vi "3-1 random controllo se compreso STOP.vi"(1 "control":bool, 2 "low limit":dbl(knob) scale=0.0..10.0 scale format="%.1f", 3 "hight limit":dbl(knob) scale=0.0..10.0 scale format="%.1f", 4 "stop":bool) -> (0 "data out":dbl(knob) scale=0.0..11.0 scale format="%.1f")   [LabVIEW 2012]
doc: "© Copyright M. Ferrari 1999"
panel:
  out "data in":dbl format="%.2f"
  # "Se control = ON, bisogna verificare che il valore sia compreso nei limiti\n                     trasferendo il valore di ingresso diviso per il range ( hight limit-low limit)\n                     in uscita; se il valore  \"data in\"  non rientra nei limiti, oppure \nse control = OFF, non viene effettuato nessun controllo e il valore di ingresso passa direttamente in uscita"
  # "Completare il VI facendo in modo che venga eseguito ciclicamente ogni 2 sec. e che \nl' esecuzione venga terminata nel caso in cui il dato in ingresso (data in) sia il doppio\ndi hight limit, oppure nel caso in cui venga premuto un apposito pulsante \"STOP\" (che \nandrˆ inserito nel pannello di controllo). Inoltre il dato di ingresso ( indicato con data in) \ndovrˆ essere generato automaticamente e risultare un valore casuale compreso fra 1 e 11"
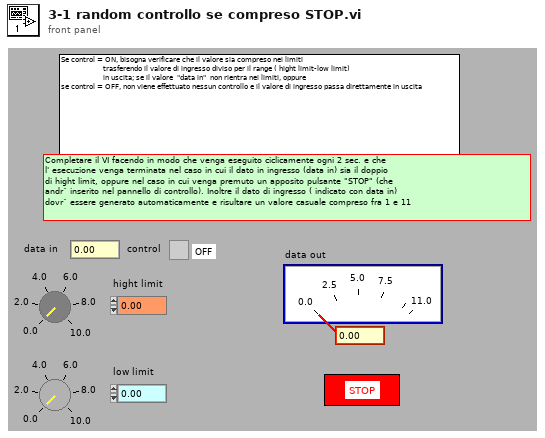
[diagram p1: front panel]
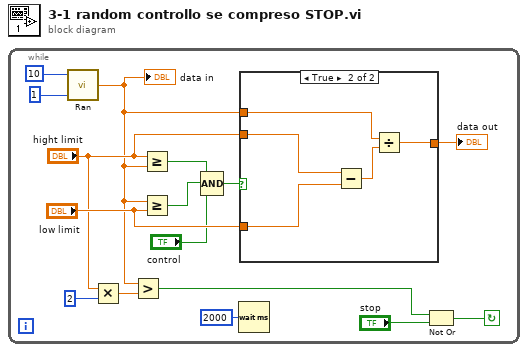
[diagram p0: block diagram]
diagram:
  n1 = while {
    stop <- w2 continue-if-true
    n2 = call "Ran.vi"("offset"=1, "mul fatt"=10) -> ("out num"=w5:dbl)  [unwired: 3 in]
    "data in" <- w5
    n3 = Multiply(x="hight limit", y=2) -> (x*y=w6:dbl)
    n4 = Greater?(x=w5, y=w6) -> (0:w4:bool)
    n5 = Greater Or Equal?(x="hight limit", y=w5) -> (x >= y?=w12:bool)
    n6 = Greater Or Equal?(x=w5, y="low limit") -> (x >= y?=w13:bool)
    n7 = Compound Arithmetic op=AND(w12, w13, "control") -> (w15:bool)
    n8 = Wait (ms)(milliseconds to wait=u32 2000) -> ()  [unwired: 1 out]
    n9 = case shown="True" w15 {
      tunnel: w5 -> [w17 w19]
      tunnel: [w17 w18] -> w11
      tunnel: "hight limit" -> [_ w21]
      tunnel: "low limit" -> [_ w20]
      frame False {
      }
      frame True {
        n10 = Subtract(x=w21, y=w20) -> (x-y=w22:dbl)
        n11 = Divide(x=w19, y=w22) -> (x/y=w18:dbl)
      }
    }
    "data out" <- w11
    n12 = Not Or(1:"stop", 2:w4) -> (0:w2:bool)
  }
